vi "from_byte_array.vi"(5 "type":refnum<class "Bytes.lvclass">, 11 "unsigned byte array":u8[](array[numeric])) -> (3 "Bytes out":refnum<class "Bytes.lvclass">)   [LabVIEW 2020, in "variant.lvlib" / "Bytes.lvclass"]
uses:
  Bytes.lvclass
  Bytes.lvclass/Bytes.ctl
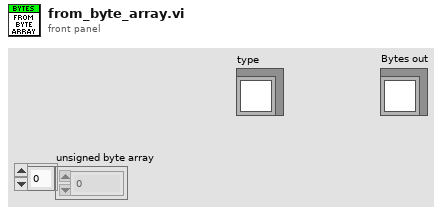
[diagram p1: front panel]
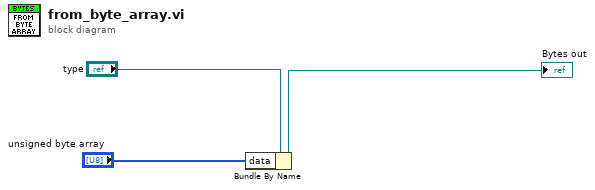
[diagram p0: block diagram]
diagram:
  n1 = Bundle By Name(cluster="type", "data"="unsigned byte array") -> (→"Bytes out":refnum<class "Bytes.lvclass">)
